vi "PH_IEEE1394Camera.set ROI Max Knob.vi"(0 "VI in":refnum<vi>, 5 "error in (no error)":errorcluster) -> (14 "VI out":refnum<vi>, 19 "error out":errorcluster)   [LabVIEW 2014, in "PH_IEEE1394Camera.lvlib"]
doc: "This VI sets several things related to ROI stuff."
uses:
  PH_IEEE1394Camera.lvlib
  PH_Basics/PH_Common/PH_Common.lvlib
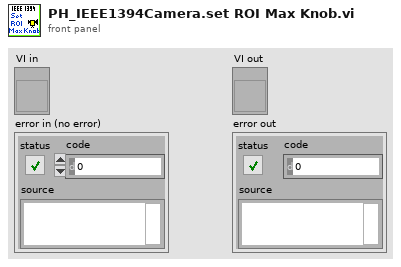
[diagram p1: front panel]
types:
  T1 = typedef "PH_IEEE1394Camera.lvlib/PH_IEEE1394Camera.i attribute.ctl" = cluster{"Gui Refs":cluster{"Brightness":refnum<vi>, "Shutter":refnum<vi>, "Gain":refnum<vi>, "Center of Gravity":refnum<vi>, "Supported Video Modes":refnum<vi>, "Trigger Polarity":refnum<vi>, "Trigger Mode":refnum<vi>, "Trigger Timeout":refnum<vi>, "Bit Depth":refnum<vi>, "Video Mode":refnum<vi>, "Top":refnum<vi>, "Bottom":refnum<vi>, "Left":refnum<vi>, "Right":refnum<vi>, "Set ROI to Maximum":refnum<vi>, "Camera Details":refnum<vi>, "Current Cam Attributes":refnum<vi>, "Attribute to set":refnum<vi>, "Num Value":refnum<vi>, "String Value":refnum<vi>, "Bool Value":refnum<vi>, "Set Cam Attribute":refnum<vi>}, "Cam":cluster{"IMAQ1394 Session":T2, "Camera Details":T3}, "Current Attributes":T4[], "Supported Video Modes ":cluster{"Video Mode":u32, "Video Mode Name":string}[], "Wanted Attributes":cluster{"Name":string, "Num Value":dbl, "String Value":string, "Boolean Value":bool}[], "Cam Attributes":T6}
  T2 = typedef "IMAQdx.ctl" = refnum<k21>
  T3 = typedef "PH_IEEE1394Camera.lvlib/PH_IEEE1394Camera.Cam Details.ctl" = cluster{"Model":string, "Serial Number":dbl, "Cam name (Machinery)":string, "Bus Type":string}
  T4 = typedef "PH_IEEE1394Camera.lvlib/PH_IEEE1394Camera.Cam Attribute.ctl" = cluster{"Information":cluster{"Type":T5, "Readable":bool, "Writable":bool, "Name":string}, "Num Value":dbl, "String Value":string, "Maximum":dbl, "Minimum":dbl, "Units":string, "Description":string, "EnumStrings[]":string[], "EnumValues[]":u32[], "Boolean Value":bool}
  T5 = typedef "NI_Vision_Acquisition_Software.lvlib/IMAQdx Attribute Type.ctl" = enum32{"U32", "I64", "DBL", "String", "Enum", "Bool", "Command"}
  T6 = typedef "PH_IEEE1394Camera.lvlib/PH_IEEE1394Camera.Relevant Cam Attributes.ctl" = cluster{"Video Mode":cluster{"Name":string, "Index":i32}, "Brightness":cluster{"Name":string, "Index":i32}, "Gain":cluster{"Name":string, "Index":i32}, "Shutter":cluster{"Name":string, "Index":i32}, "Trigger Pol":cluster{"Name":string, "Index":i32}, "Trigger Mode":cluster{"Name":string, "Index":i32}, "Timeout":cluster{"Name":string, "Index":i32}, "Bit Depth":cluster{"Name":string, "Index":i32}, "Pixel Bits":cluster{"Name":string, "Index":i32}, "Pixel Bytes":cluster{"Name":string, "Index":i32}, "Left":cluster{"Name":string, "Index":i32}, "Right":cluster{"Name":string, "Index":i32}, "Top":cluster{"Name":string, "Index":i32}, "Bottom":cluster{"Name":string, "Index":i32}}
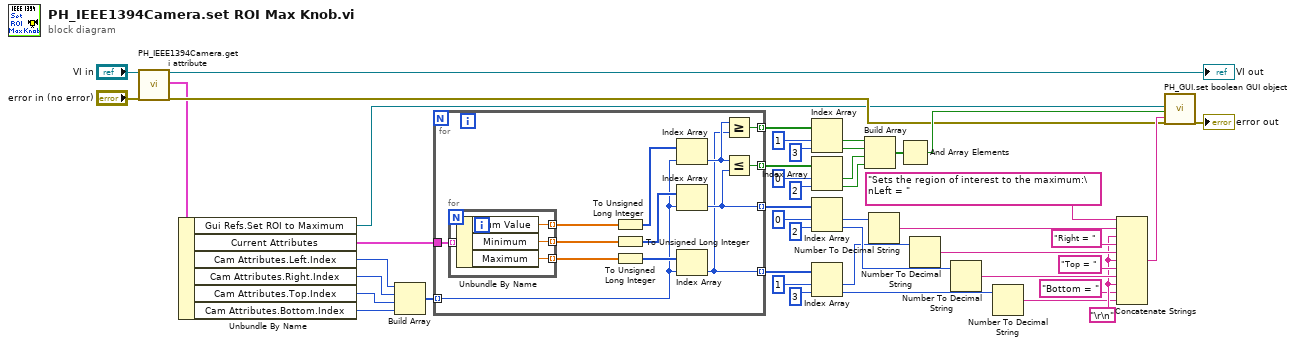
[diagram p0: block diagram]
diagram:
  w35 = "\r\n"
  n1 = call "PH_IEEE1394Camera.get i attribute.vi"("i ref in"="VI in", "error in (no error)"="error in (no error)") -> ("i ref out"=→"VI out":refnum<vi>, "i attribute"=w29:T1, "error out"=w30:errorcluster)  [unwired: 15 in]
  n2 = Unbundle By Name(w29) -> ("Gui Refs.Set ROI to Maximum"=w28:refnum<vi>, "Current Attributes"=w27:T4[], "Cam Attributes.Left.Index"=w23:i32, "Cam Attributes.Right.Index"=w24:i32, "Cam Attributes.Top.Index"=w25:i32, "Cam Attributes.Bottom.Index"=w26:i32)
  n3 = Build Array(w23, w24, w25, w26) -> (w22:i32[])
  n4 = for {
    tunnel: w27 -> [w58]
    tunnel: w22 -> [w46] mode=indexing
    tunnel: [w49] -> w15 mode=indexing
    tunnel: [w50] -> w21 mode=indexing
    tunnel: [w48] -> w6 mode=indexing
    tunnel: [w47] -> w7 mode=indexing
    n5 = for {
      tunnel: w58 -> [w62] mode=indexing
      tunnel: [w61] -> w56 mode=indexing
      tunnel: [w60] -> w55 mode=indexing
      tunnel: [w59] -> w57 mode=indexing
      n6 = Unbundle By Name(w62) -> ("Num Value"=w59:dbl, "Minimum"=w61:dbl, "Maximum"=w60:dbl)
    }
    n7 = To Unsigned Long Integer(number=w57) -> (unsigned 32bit integer=w52:u32[])
    n8 = To Unsigned Long Integer(number=w56) -> (unsigned 32bit integer=w54:u32[])
    n9 = To Unsigned Long Integer(number=w55) -> (unsigned 32bit integer=w53:u32[])
    n10 = Index Array(array=w52, index=w46) -> (element=w51:u32)
    n11 = Index Array(array=w54, index=w46) -> (element=w50:u32)
    n12 = Index Array(array=w53, index=w46) -> (element=w49:u32)
    n13 = Greater Or Equal?(x=w51, y=w49) -> (x >= y?=w47:bool)
    n14 = Less Or Equal?(x=w51, y=w50) -> (x <= y?=w48:bool)
  }
  n15 = Index Array(array=w7, index #1=1 ("index"), index #2=3 ("index")) -> (element #1=w5:bool, element #2=w4:bool)
  n16 = Index Array(array=w6, index #1=0 ("index"), index #2=2 ("index")) -> (element #1=w3:bool, element #2=w2:bool)
  n17 = Index Array(array=w21, index #1=0 ("index"), index #2=2 ("index")) -> (element #1=w12:u32, element #2=w18:u32)
  n18 = Index Array(array=w15, index #1=1 ("index"), index #2=3 ("index")) -> (element #1=w14:u32, element #2=w13:u32)
  n19 = Build Array(w5, w4, w3, w2) -> (w1:bool[])
  n20 = Number To Decimal String(number=w12) -> (decimal integer string=w40:string)  [unwired: 1 in]
  n21 = And Array Elements(Boolean array=w1) -> (logical AND=w43:bool)
  n22 = Number To Decimal String(number=w14) -> (decimal integer string=w38:string)  [unwired: 1 in]
  n23 = Number To Decimal String(number=w18) -> (decimal integer string=w36:string)  [unwired: 1 in]
  n24 = Number To Decimal String(number=w13) -> (decimal integer string=w33:string)  [unwired: 1 in]
  n25 = Concatenate Strings("Sets the region of interest to the maximum:\nLeft = " ("Tip Strip"), w40, w35, "Right = " ("string"), w38, w35, "Top = " ("string"), w36, w35, "Bottom = " ("string"), w33) -> (w41:string)
  n26 = call "PH_GUI.set boolean GUI object.vi"("Boolean Knob GUI Ref"=w28, "Value"=w43, "error in (no error)"=w30, "Tip Strip"=w41) -> ("error out"=→"error out":errorcluster)  [unwired: 15 in]
